vi "create log file.vi"(8 "error in (no error)":errorcluster, 11 "Socket in":refnum<class "Socket.lvclass">) -> (0 "error out":errorcluster, 3 "Socket out":refnum<class "Socket.lvclass">)   [LabVIEW 2018, in "Socket.lvclass"]
uses:
  Socket.lvclass
  Socket.lvclass/Socket.ctl
  Log File/CM_Log File.lvclass/CM_Log File.ctl
  Log File/CM_Log File.lvclass
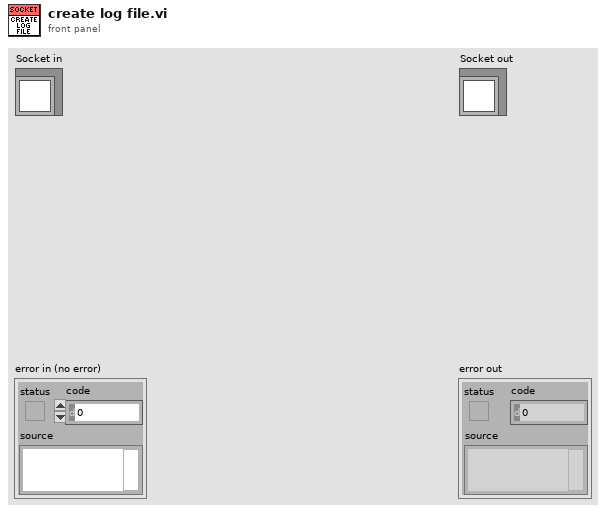
[diagram p1: front panel]
types:
  T1 = typedef "LVDateTimeRec.ctl" = cluster{"fractional second":dbl, "second":i32, "minute":i32, "hour":i32, "day of month":i32, "month":i32, "year":i32, "day of week":i32, "day of year":i32, "DST":i32}
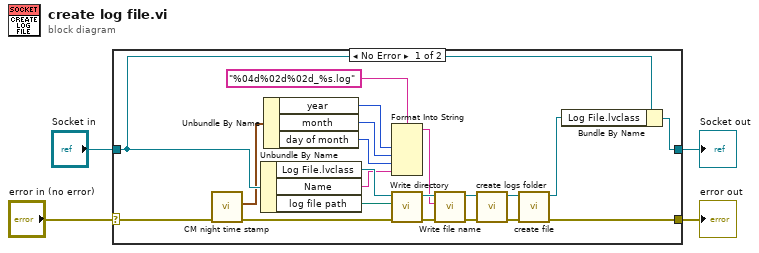
[diagram p0: block diagram]
diagram:
  n1 = case shown="No Error" "error in (no error)" {
    selector: "error in (no error)" -> [w14 w27]
    tunnel: [w19 w27] -> w3
    tunnel: [w23 w26] -> w1
    tunnel: "Socket in" -> [w24 w26]
    frame No Error {
      n2 = call "CM night time stamp.vi"("error in (no error)"=w14) -> ("error out"=w13:errorcluster, "date time rec"=w8:T1)  [unwired: 9 in]
      n3 = Unbundle By Name(w24) -> ("Log File.lvclass"=w25:refnum<class "CM_Log File.lvclass">, "Name"=w6:string, "log file path"=w5:path)
      n4 = Unbundle By Name(w8) -> ("year"=w12:i32, "month"=w11:i32, "day of month"=w10:i32)
      n5 = Format Into String(format string="%04d%02d%02d_%s.log", w12, w11, w10, w6) -> (resulting string=w7:string)  [unwired: 2 in, 1 out]
      n6 = call "Write directory.vi"("error in (no error)"=w13, "directory"=w5, "Log File in"=w25) -> ("error out"=w16:errorcluster, "Log File out"=w18:refnum<class "CM_Log File.lvclass">)  [unwired: 7 in]
      n7 = call "Write file name.vi"("error in (no error)"=w16, "file name"=w7, "Log File in"=w18) -> ("error out"=w15:errorcluster, "Log File out"=w17:refnum<class "CM_Log File.lvclass">)  [unwired: 7 in]
      n8 = call "create logs folder.vi"("error in (no error)"=w15, "Log File in"=w17) -> ("error out"=w20:errorcluster, "Log File out"=w22:refnum<class "CM_Log File.lvclass">)  [unwired: 8 in]
      n9 = call "create file.vi"("error in (no error)"=w20, "Log File in"=w22) -> ("error out"=w19:errorcluster, "Log File out"=w21:refnum<class "CM_Log File.lvclass">)  [unwired: 8 in]
      n10 = Bundle By Name(cluster=w24, "Log File.lvclass"=w21) -> (w23:refnum<class "Socket.lvclass">)
    }
    frame Error {
    }
  }
  "error out" <- w3
  "Socket out" <- w1
